vi "Rohde & Schwarz VNA Read Start and Stop Frequencies.vi"(6 "Channel":i8=1 min=1 max=99 step=1, 7 "Rohde & Schwarz VNA":T1, 8 "error in (no error)":errorcluster, 11 "VISA Resource Name":refnum<visa-resource-name>) -> (0 "error out":errorcluster, 2 "Start/Stop Freqs, MHz":cluster{"Fstart":dbl, "Fstop":dbl}[](array[cluster]), 3 "dup VISA Resource Name":refnum<visa-resource-name>)   [LabVIEW 2011]
doc: "This VI for the HP8753B Network Analyzers reads the stimulus values. Except when performing log sweeps and freq list sweeps, this VI uses the start and stop values and the number of points to calcuate the stimulus values."
uses:
  TypeDefs/Rohde & Schwarz VNA Instrument Info.ctl
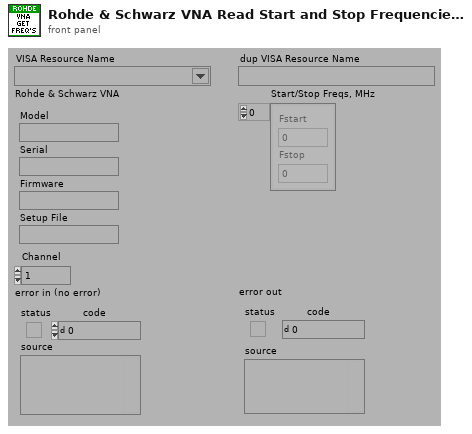
[diagram p1: front panel]
types:
  T1 = typedef "Rohde & Schwarz VNA Instrument Info.ctl" = cluster{"Model":string, "Serial":string, "Firmware":string, "Setup File":string}
  T2 = typedef "Rohde & Schwarz VNA Sweep Type.ctl" = enum32{"Linear", "Logarithmic", "Segmented", "Power", "Time", "CW"}
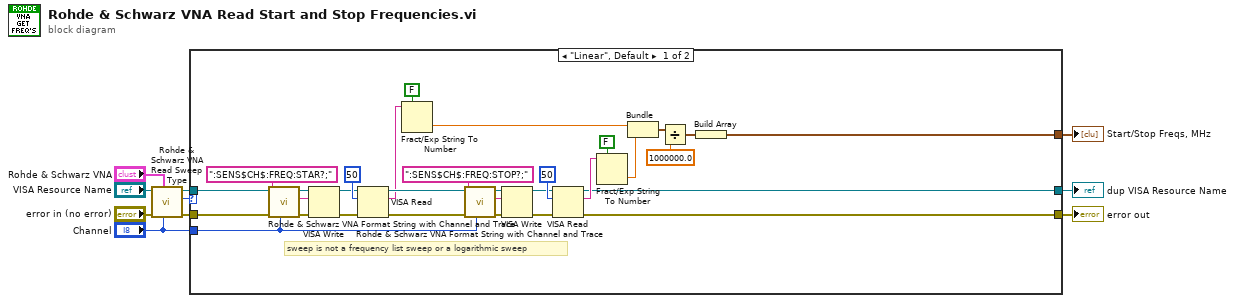
[diagram p0: block diagram]
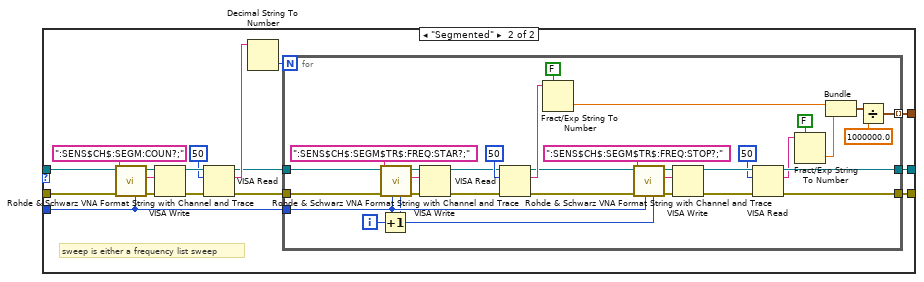
[diagram p2: hidden frame]
diagram:
  n1 = call "Rohde & Schwarz VNA Read Sweep Type.vi"("Channel"="Channel", "Rohde & Schwarz VNA"="Rohde & Schwarz VNA", "error in (no error)"="error in (no error)", "VISA Resource Name"="VISA Resource Name") -> ("error out"=w5:errorcluster, "Sweep Type"=w8:T2, "dup VISA Resource Name"=w6:refnum<visa-resource-name>)  [unwired: 1 in, 4 out]
  n2 = case shown="\"Linear\", Default" w8 {
    tunnel: w6 -> [w24 w48]
    tunnel: w5 -> [w23 w47]
    tunnel: [w31 w38] -> w10
    tunnel: [w22 w44] -> w4
    tunnel: [w16 w39] -> w3
    tunnel: "Channel" -> [w13 w40]
    frame "Linear", Default {
      # "sweep is not a frequency list sweep or a logarithmic sweep"
      n3 = call "Rohde & Schwarz VNA Format String with Channel and Trace.vi"("Channel"=w13, "String"=":SENS$CH$:FREQ:STAR?;") -> ("String Out"=w15:string)  [unwired: 1 in, 6 out]
      n4 = VISA Write(VISA resource name=w24, write buffer=w15, error in (no error)=w23) -> (VISA resource name out=w27:refnum<visa-resource-name>, error out=w37:errorcluster)  [unwired: 1 out]
      n5 = VISA Read(VISA resource name=w27, byte count=u32 50, error in (no error)=w37) -> (VISA resource name out=w35:refnum<visa-resource-name>, read buffer=w33:string, error out=w34:errorcluster)  [unwired: 1 out]
      n6 = Fract/Exp String To Number(use system decimal point (T)=FALSE, string=w33) -> (number=w20:dbl)  [unwired: 3 out]
      n7 = call "Rohde & Schwarz VNA Format String with Channel and Trace.vi"("Channel"=w13, "String"=":SENS$CH$:FREQ:STOP?;") -> ("String Out"=w14:string)  [unwired: 1 in, 6 out]
      n8 = VISA Write(VISA resource name=w35, write buffer=w14, error in (no error)=w34) -> (VISA resource name out=w28:refnum<visa-resource-name>, error out=w36:errorcluster)  [unwired: 1 out]
      n9 = VISA Read(VISA resource name=w28, byte count=u32 50, error in (no error)=w36) -> (VISA resource name out=w16:refnum<visa-resource-name>, read buffer=w32:string, error out=w31:errorcluster)  [unwired: 1 out]
      n10 = Fract/Exp String To Number(use system decimal point (T)=FALSE, string=w32) -> (number=w19:dbl)  [unwired: 3 out]
      n11 = Bundle(w20, w19) -> (w18:cluster{dbl, dbl})  [unwired: 1 out]
      n12 = Divide(x=w18, y=1000000.0) -> (x/y=w17:cluster{dbl, dbl})
      n13 = Build Array(w17) -> (w22:cluster{dbl, dbl}[])
    }
    frame "Segmented" {
      # "sweep is either a frequency list sweep"
      n14 = call "Rohde & Schwarz VNA Format String with Channel and Trace.vi"("Trace"=w40, "String"=":SENS$CH$:SEGM:COUN?;") -> ("String Out"=w50:string)  [unwired: 1 in, 6 out]
      n15 = VISA Write(VISA resource name=w48, write buffer=w50, error in (no error)=w47) -> (VISA resource name out=w51:refnum<visa-resource-name>, error out=w52:errorcluster)  [unwired: 1 out]
      n16 = VISA Read(VISA resource name=w51, byte count=u32 50, error in (no error)=w52) -> (VISA resource name out=w43:refnum<visa-resource-name>, read buffer=w45:string, error out=w42:errorcluster)  [unwired: 1 out]
      n17 = Decimal String To Number(string=w45) -> (number=w41:i32)  [unwired: 1 in, 2 out]
      n18 = for {
        N: w41 -> [_]
        tunnel: [w69] -> w44 mode=indexing
        tunnel: w43 -> [w76]
        tunnel: w42 -> [w75]
        tunnel: w40 -> [w55]
        tunnel: [w57] -> w39
        tunnel: [w56] -> w38
        i -> [w65]
        n19 = Increment(x=w65) -> (x+1=w54:i32)
        n20 = call "Rohde & Schwarz VNA Format String with Channel and Trace.vi"("Trace"=w54, "Channel"=w55, "String"=":SENS$CH$:SEGM$TR$:FREQ:STAR?;") -> ("String Out"=w78:string)  [unwired: 6 out]
        n21 = VISA Write(VISA resource name=w76, write buffer=w78, error in (no error)=w75) -> (VISA resource name out=w77:refnum<visa-resource-name>, error out=w74:errorcluster)  [unwired: 1 out]
        n22 = VISA Read(VISA resource name=w77, byte count=u32 50, error in (no error)=w74) -> (VISA resource name out=w58:refnum<visa-resource-name>, read buffer=w66:string, error out=w59:errorcluster)  [unwired: 1 out]
        n23 = Fract/Exp String To Number(use system decimal point (T)=FALSE, string=w66) -> (number=w67:dbl)  [unwired: 3 out]
        n24 = call "Rohde & Schwarz VNA Format String with Channel and Trace.vi"("Trace"=w54, "Channel"=w55, "String"=":SENS$CH$:SEGM$TR$:FREQ:STOP?;") -> ("String Out"=w62:string)  [unwired: 6 out]
        n25 = VISA Write(VISA resource name=w58, write buffer=w62, error in (no error)=w59) -> (VISA resource name out=w63:refnum<visa-resource-name>, error out=w64:errorcluster)  [unwired: 1 out]
        n26 = VISA Read(VISA resource name=w63, byte count=u32 50, error in (no error)=w64) -> (VISA resource name out=w57:refnum<visa-resource-name>, read buffer=w53:string, error out=w56:errorcluster)  [unwired: 1 out]
        n27 = Fract/Exp String To Number(use system decimal point (T)=FALSE, string=w53) -> (number=w71:dbl)  [unwired: 3 out]
        n28 = Bundle(w67, w71) -> (w70:cluster{dbl, dbl})  [unwired: 1 out]
        n29 = Divide(x=w70, y=1000000.0) -> (x/y=w69:cluster{dbl, dbl})
      }
    }
  }
  "dup VISA Resource Name" <- w3
  "error out" <- w10
  "Start/Stop Freqs, MHz" <- w4
